vi "_FPGA Wait Serial.vi"(4 "error in":errorcluster, 5 "Timeout (2000ms)":u32=2000, 6 "Indicator":T1=enum."SendSerial") -> (0 "error out":errorcluster)   [LabVIEW 2012]
uses:
  Type/_FPGA Indicator.ctl
  Type/_LED States.ctl
  _RT Global.vi
  <vilib>/Utility/error.llb/Error Cluster From Error Code.vi
  <vilib>/rvi/errors/niLvFpgaAdjustHostInterfaceError.vi
  <vilib>/rvi/interface/nirviReadWriteControl/nirviReadWriteControl.xnode
  FPGA Bitfiles/FPGA9602.lvbitx
  NiFpgaLv.dll
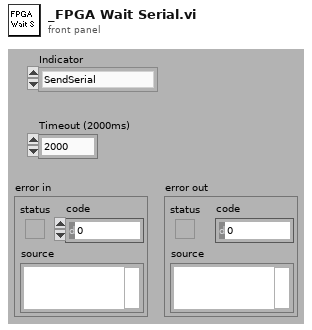
[diagram p1: front panel]
types:
  T1 = typedef "_FPGA Indicator.ctl" = enum16{"Done", "Ready", "Count Available", "SendSerial", "LED State"}
  T2 = typedef "_LED States.ctl" = enum8{"Idle", "Solid B", "Solid R", "Solid P", "Off B", "Off R", "Off P", "Off BRP", "Off RP", "Flash R&P", "Flash P"}
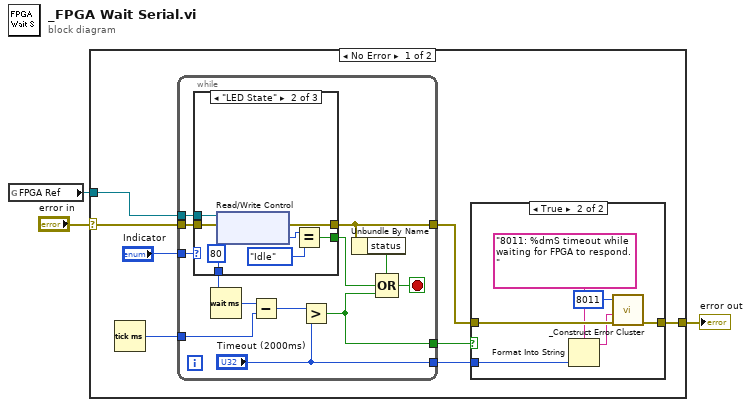
[diagram p0: block diagram]
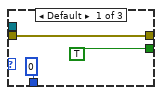
[diagram p3: hidden frame]
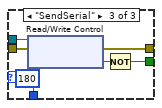
[diagram p4: hidden frame]
diagram:
  n1 = global read "_RT Global.vi" "FPGA Ref"() -> (w1:refnum<k20>)
  n2 = case shown="No Error" "error in" {
    selector: "error in" -> [w6 w47]
    tunnel: [w8 w47] -> w3
    tunnel: w1 -> [w4 _]
    frame No Error {
      n3 = Tick Count (ms)() -> (millisecond timer value=w11:u32)
      n4 = while {
        tunnel: w4 -> [w30]
        tunnel: w6 -> [w29]
        tunnel: [w21] -> w9
        tunnel: w11 -> [w28]
        tunnel: [w24] -> w10
        tunnel: "Indicator" -> [w23]
        tunnel: ["Timeout (2000ms)"] -> w5
        stop <- w25 stop-if-true
        n5 = case shown="\"LED State\"" w23 {
          tunnel: w30 -> [_ w40 w46]
          tunnel: w29 -> [w32 w39 w45]
          tunnel: [w32 w38 w44] -> w21
          tunnel: [TRUE w37 w42] -> w26
          tunnel: [u32 0 ("milliseconds to wait") u32 80 ("milliseconds to wait") u32 180 ("milliseconds to wait")] -> w18
          frame Default {
          }
          frame "LED State" {
            n6 = xnode "Read/Write Control"("FPGA VI Reference In"=w40, "error in"=w39) -> ("error out"=w38:errorcluster, "LED States"=w36:T2)  [unwired: 1 out]
            n7 = Equal?(x=w36, y=_LED_States."Idle" ("R/W Status")) -> (x = y?=w37:bool)
          }
          frame "SendSerial" {
            n8 = xnode "Read/Write Control"("FPGA VI Reference In"=w46, "error in"=w45) -> ("error out"=w44:errorcluster, "Send Serial"=w43:bool)  [unwired: 1 out]
            n9 = Not(x=w43) -> (.not. x?=w42:bool)
          }
        }
        n10 = Wait (ms)(milliseconds to wait=w18) -> (millisecond timer value=w19:u32)
        n11 = Subtract(x=w19, y=w28) -> (x-y=w27:u32)
        n12 = Greater?(x=w27, y="Timeout (2000ms)") -> (0:w24:bool)
        n13 = Unbundle By Name(w21) -> ("status"=w20:bool)
        n14 = Compound Arithmetic op=OR(w20, w26, w24) -> (w25:bool)
      }
      n15 = case shown="True" w10 {
        tunnel: w9 -> [_ w17]
        tunnel: [_ w16] -> w8
        tunnel: w5 -> [_ w13]
        frame False {
        }
        frame True {
          n16 = Format Into String(format string="8011: %dmS timeout while waiting for FPGA to respond.", w13) -> (resulting string=w14:string)  [unwired: 2 in, 1 out]
          n17 = call "_Construct Error Cluster.vi"("error in"=w17, "reason"=w14, "errorCode"=8011) -> ("error out"=w16:errorcluster)  [unwired: 1 in, 3 out]
        }
      }
    }
    frame Error {
    }
  }
  "error out" <- w3
